vi "Save Para Setting UI.vi"() -> ()   [LabVIEW 2016]
uses:
  <vilib>/Utility/error.llb/DialogType.ctl
  Architecture/Queue Management/ARC_Queue Create_Single.vi
  Architecture/Queue Management/ARC_Queue Insert Element.vi
  Architecture/Queue Management/ARC_Queue Remove Element.vi
  Architecture/Queue Management/ARC_Queue Destroy_Single.vi
panel:
  in  "Parameter":cluster{"Q-Local":string, "Variant":variant}
  in  "Tab Control":enum32{"Page 1"}(tab)
  in  "AutoInterval":i32=1 caption="自动挑点时间间隔：" min=1 max=1000 step=1
  out "info":string
  in  "FileNote":string caption="文件备注："
  in  "FileName":string caption="文件名："
  in  "CFilePath":path caption="文件夹路径："
  in  "OK":bool
  out "error out":errorcluster caption="错误输出"
  # "文件存储设置"
  # "s"
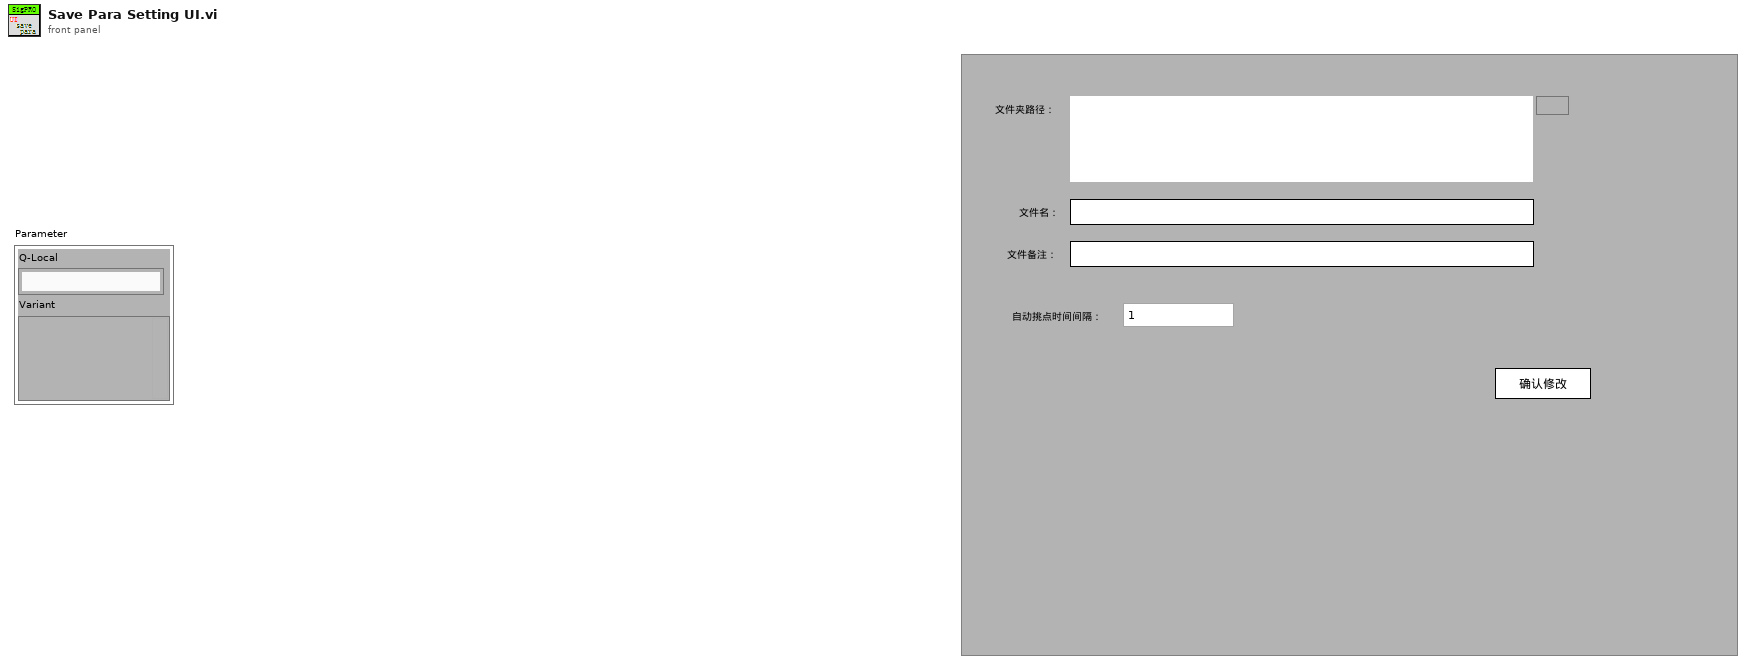
[diagram p1: front panel]
types:
  T1 = cluster{"error":errorcluster, "Event":string, "Data":variant, "Q_Local":string, "Caller":string, "Refs":cluster{"ContiousFileName":refnum<vi>, "SelectFileName":refnum<vi>, "CFilePath":refnum<vi>, "SFilePath":refnum<vi>}, "States":cluster{"CExist?":bool, "SExist?":bool}, "ContinuousFile？":bool}
  T2 = enum16{"open", "replace", "create", "open or create", "replace or create", "replace or create with confirmation"}
  T3 = typedef "DialogType.ctl" = u16
  T4 = typedef "Global para Config.ctl" = cluster{"Timing":cluster{"SampleRate":i32}, "SavePara":cluster{"FlowDiskMode":T5, "SelectMode":T6, "FolderPath":path, "Filename":string, "FileNote":string, "AutoInterval":i32, "Template":path}, "ConfigDS Path*":path, "Tdms Ref*":refnum<k34>}
  T5 = typedef "File Save Mode.ctl" = i32
  T6 = typedef "Select Point Mode.ctl" = i32
  T7 = cluster{"DfltDataFolder":path, "ParaFolder":path, "SysCfg":path, "CHdef":path, "ModCfg":path, "DT Folder":path, "ErrorLog":path, "HBMlic":path, "HBMDriver":path}
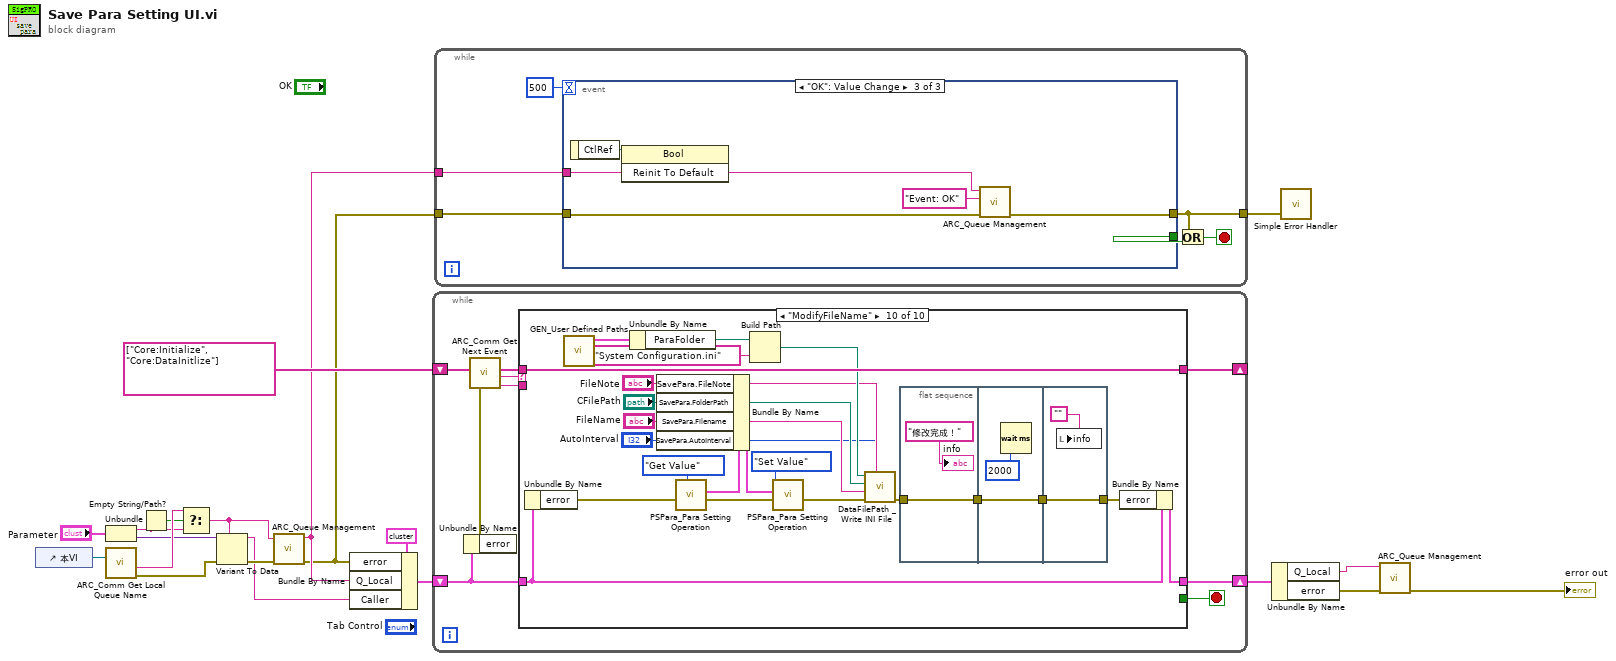
[diagram p0: block diagram]
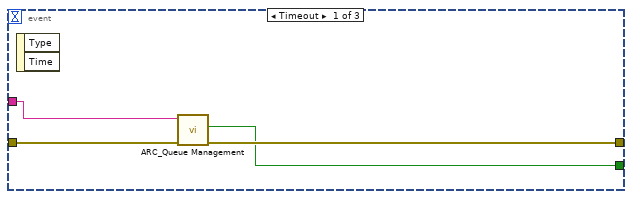
[diagram p2: hidden frame]
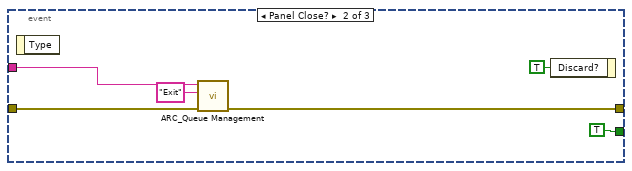
[diagram p3: hidden frame]
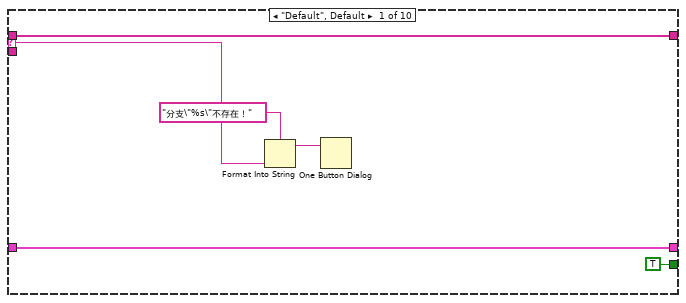
[diagram p4: hidden frame]
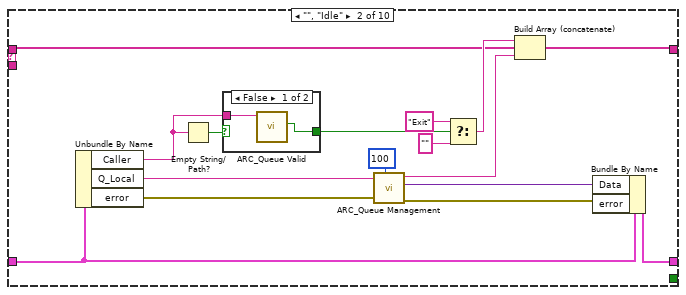
[diagram p5: hidden frame]
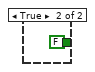
[diagram p6: hidden frame]
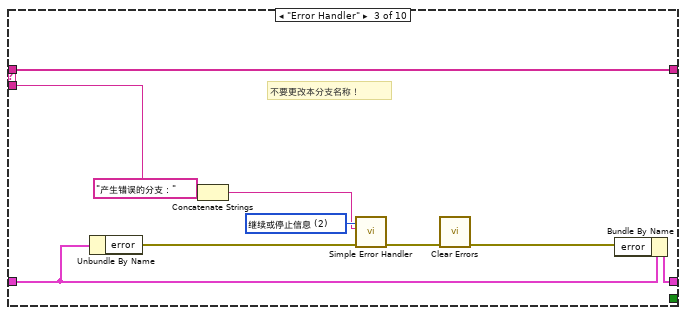
[diagram p7: hidden frame]
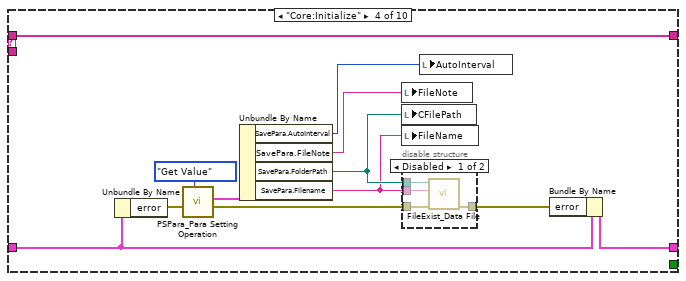
[diagram p8: hidden frame]
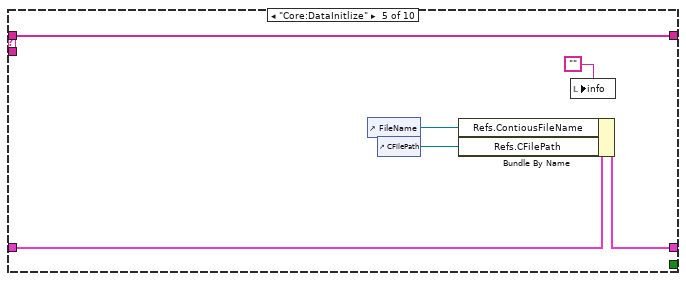
[diagram p10: hidden frame]
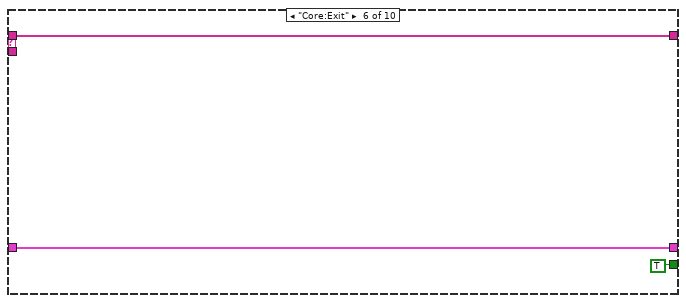
[diagram p11: hidden frame]
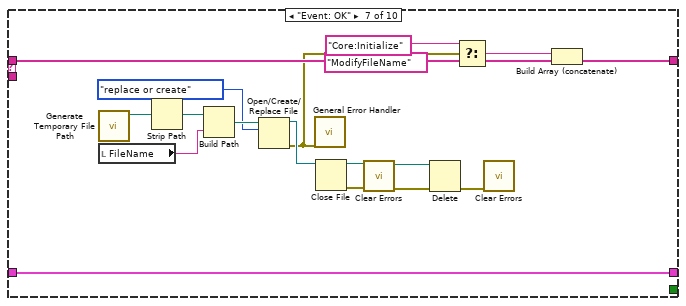
[diagram p12: hidden frame]
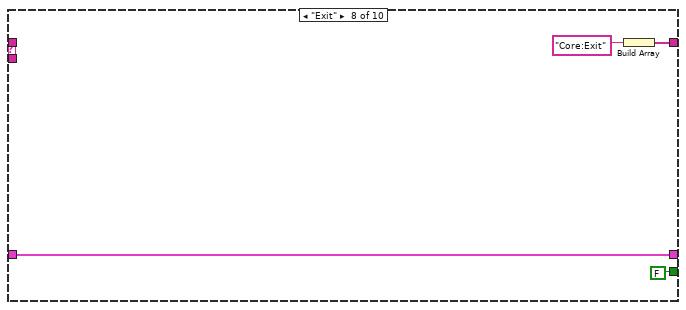
[diagram p13: hidden frame]
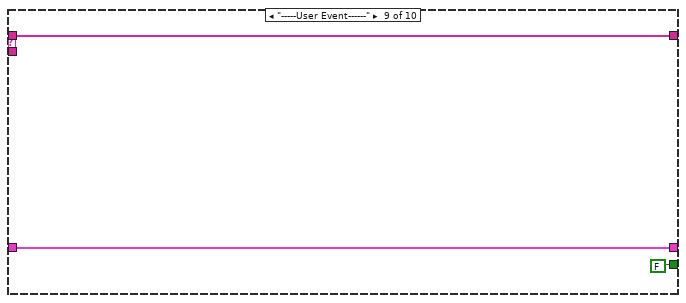
[diagram p14: hidden frame]
diagram:
  n1 = control-ref of="本VI"() -> (w6:refnum<vi>)
  n2 = Unbundle("Parameter") -> ("Q-Local"=w8:string, "Variant"=w11:variant)
  n3 = call "ARC_Comm Get Local Queue Name.vi"("VI Ref"=w6) -> ("error out"=w7:errorcluster, "VI  Name"=w12:string)  [unwired: 8 in, 1 out]
  n4 = Empty String/Path?(string/path=w8) -> (empty?=w10:bool)
  n5 = Select(t=w12, s=w10, f=w8) -> (s? t:f=w2:string)
  n6 = Variant To Data(error in=w7, type=w2, Variant=w11) -> (data=w1:string, error out=w5:errorcluster)
  n7 = call-poly "ARC_Queue Management.vi"("error in"=w5, "Queue Name"=w2) -> ("error out"=w3:errorcluster, "Queue Name dup"=w4:string)  [unwired: 7 in, 1 out]
  n8 = Bundle By Name(cluster=T1 {"error"={"status"=FALSE, "code"=0, "source"=""}, "Event"="", "Data"=variant, "Q_Local"="", "Caller"="", "Refs"={"ContiousFileName"=refnum, "SelectFileName"=refnum, "CFilePath"=refnum, "SFilePath"=refnum}, "States"={"CExist?"=FALSE, "SExist?"=FALSE}, "ContinuousFile？"=FALSE} ("TmpData"), "error"=w3, "Q_Local"=w4, "Caller"=w1) -> (w16:T1)
  n9 = while {
    shift-right: [w26] -> w19
    shift-left: w16 -> [w27]
    shift-right: [w25] -> _
    shift-left: string[] ["Core:Initialize", "Core:DataInitlize"] ("event queue out") -> [w21]
    stop <- w29 stop-if-true
    n10 = Unbundle By Name(w27) -> ("error"=w28:errorcluster)
    n11 = call "ARC_Comm Get Next Event.vi"("error in (no error)"=w28, "event queue in"=w21) -> ("prev event"=w24:string, "next event"=w22:string, "event queue out"=w23:string[])  [unwired: 4 in]
    n12 = case shown="\"ModifyFileName\"" w22 {
      selector: w22 -> [w33 _ _ _ _ _ _ _ _ _]
      tunnel: w23 -> [w34 w37 w64 w76 w87 w88 w106 _ w112 w132]
      tunnel: w24 -> [_ _ w55 _ _ _ _ _ _ _]
      tunnel: [TRUE _ _ _ _ TRUE _ FALSE FALSE _] -> w29
      tunnel: w27 -> [w35 w47 w60 w74 w86 w89 w107 w110 w113 w131]
      tunnel: [w35 w50 w59 w71 w85 w89 w107 w110 w113 w129] -> w26
      tunnel: [w34 w48 w64 w76 w87 w88 w105 w108 w112 w132] -> w25
      frame "Default", Default {
        n13 = Format Into String(format string="分支\"%s\"不存在！" ("格式字符串"), w33) -> (resulting string=w32:string)  [unwired: 2 in, 1 out]
        n14 = One Button Dialog(message=w32) -> ()  [unwired: 1 in, 1 out]
      }
      frame "", "Idle" {
        n15 = Unbundle By Name(w47) -> ("Caller"=w41:string, "Q_Local"=w46:string, "error"=w45:errorcluster)
        n16 = Empty String/Path?(string/path=w41) -> (empty?=w44:bool)
        n17 = case shown="False" w44 {
          tunnel: [w52 FALSE ("Not Exist?")] -> w43
          tunnel: w41 -> [w53 _]
          frame False {
            n18 = call "ARC_Queue Valid.vi"("Queue Name(unamed)"=w53) -> ("Not Exist?"=w52:bool)  [unwired: 8 in, 2 out]
          }
          frame True {
          }
        }
        n19 = call-poly "ARC_Queue Management.vi"("Time out(-1)_queue out"=100 ("Time out(-1)"), "error in (no error)"=w45, "Queue Name(unamed)"=w46) -> ("error out"=w51:errorcluster, "Data"=w49:variant, "Event"=w40:string)  [unwired: 5 in, 1 out]
        n20 = Select(t="Exit" ("Event"), s=w43, f="") -> (s? t:f=w38:string)
        n21 = Build Array (concatenate)(w38, w37, w40) -> (w48:string[])
        n22 = Bundle By Name(cluster=w47, "Data"=w49, "error"=w51) -> (w50:T1)
      }
      frame "Error Handler" {
        w58 = T3 2 items=["无对话框", "确定信息", "继续或停止信息", "确定信息＋警告", "继续/停止+警告"] ("type of dialog (OK msg:1)")
        # "不要更改本分支名称！"
        n23 = Unbundle By Name(w60) -> ("error"=w61:errorcluster)
        n24 = Concatenate Strings("产生错误的分支：" ("字符串"), w55) -> (w57:string)
        n25 = call <vilib>:"Simple Error Handler.vi"("error source (\" \")"=w57, "type of dialog (OK msg:1)"=w58, "error in (no error)"=w61) -> ("error out"=w62:errorcluster)  [unwired: 2 in, 4 out]
        n26 = call <vilib>:"Clear Errors.vi"("error in (no error)"=w62) -> ("error out"=w63:errorcluster)  [unwired: 5 in, 1 out]
        n27 = Bundle By Name(cluster=w60, "error"=w63) -> (w59:T1)
      }
      frame "Core:Initialize" {
        n28 = Unbundle By Name(w74) -> ("error"=w73:errorcluster)
        n29 = call "PSPara_Para Setting Operation.vi"("Operation"=enum16{"Set Value", "Get Value", "Initialize"}."Get Value", "error in"=w73) -> ("error out"=w70:errorcluster, "_Para"=w72:T4)  [unwired: 8 in]
        n30 = Unbundle By Name(w72) -> ("SavePara.AutoInterval"=w65:i32, "SavePara.FileNote"=w66:string, "SavePara.FolderPath"=w68:path, "SavePara.Filename"=w67:string)
        n31 = local write "FileNote"(w66) -> ()
        n32 = local write "CFilePath"(w68) -> ()
        n33 = local write "FileName"(w67) -> ()
        n34 = disable-structure shown="Disabled" {
          disable-tunnel: w70 -> [w80 w81]
          disable-tunnel: [w79 w81] -> w69
          disable-tunnel: w68 -> [w78 _]
          disable-tunnel: w67 -> [w77 _]
          frame Disabled {
            n35 = call "FileExist_Data File.vi"("error in"=w80, "Filename"=w77, "FolderPath"=w78) -> ("error out"=w79:errorcluster)  [unwired: 7 in, 1 out]
          }
          frame Enabled {
          }
        }
        n36 = local write "AutoInterval"(w65) -> ()
        n37 = Bundle By Name(cluster=w74, "error"=w69) -> (w71:T1)
      }
      frame "Core:DataInitlize" {
        n38 = control-ref of="FileName"() -> (w84:refnum<vi>)
        n39 = control-ref of="CFilePath"() -> (w83:refnum<vi>)
        n40 = Bundle By Name(cluster=w86, "Refs.ContiousFileName"=w84, "Refs.CFilePath"=w83) -> (w85:T1)
        n41 = local write "info"("") -> ()
      }
      frame "Core:Exit" {
      }
      frame "Event: OK" {
        n42 = call <vilib>:"Generate Temporary File Path.vi"() -> ("Unique Temporary File Path"=w101:path)  [unwired: 10 in, 1 out]
        n43 = local read "FileName"() -> (w104:string)
        n44 = Strip Path(path=w101) -> (stripped path=w91:path)  [unwired: 1 out]
        n45 = Build Path(base path=w91, name or relative path=w104) -> (appended path=w103:path)
        n46 = Open/Create/Replace File(file path (use dialog)=w103, operation (0:open)=T2."replace or create" ("操作(0:open)")) -> (refnum out=w100:refnum<file>, error out=w95:errorcluster)  [unwired: 4 in, 1 out]
        n47 = call <vilib>:"General Error Handler.vi"("error in (no error)"=w95) -> ()  [unwired: 10 in, 5 out]
        n48 = Close File(refnum=w100) -> (path=w99:path, error out=w98:errorcluster)  [unwired: 1 in]
        n49 = call <vilib>:"Clear Errors.vi"("error in (no error)"=w98) -> ("error out"=w97:errorcluster)  [unwired: 5 in, 1 out]
        n50 = Delete(path (use dialog)=w99, error in=w97) -> (error out=w96:errorcluster)  [unwired: 3 in, 2 out]
        n51 = Select(t="Core:Initialize", s=w95, f="ModifyFileName") -> (s? t:f=w92:string)
        n52 = call <vilib>:"Clear Errors.vi"("error in (no error)"=w96) -> ()  [unwired: 5 in, 2 out]
        n53 = Build Array (concatenate)(w92, w106) -> (w105:string[])
      }
      frame "Exit" {
        n54 = Build Array("Core:Exit" ("Remaining States")) -> (w108:string[])
      }
      frame "-----User Event------" {
      }
      frame "ModifyFileName" {
        n55 = Unbundle By Name(w131) -> ("error"=w130:errorcluster)
        n56 = call "GEN_User Defined Paths.vi"() -> ("UserDefinedPath"=w124:T7)  [unwired: 11 in]
        n57 = Unbundle By Name(w124) -> ("ParaFolder"=w123:path)
        n58 = call "PSPara_Para Setting Operation.vi"("Operation"=enum16{"Set Value", "Get Value", "Initialize"}."Get Value", "error in"=w130) -> ("error out"=w128:errorcluster, "_Para"=w134:T4)  [unwired: 8 in]
        n59 = Bundle By Name(cluster=w134, "SavePara.FileNote"="FileNote", "SavePara.FolderPath"="CFilePath", "SavePara.Filename"="FileName", "SavePara.AutoInterval"="AutoInterval") -> (w133:T4)
        n60 = Build Path(base path=w123, name or relative path="System Configuration.ini") -> (appended path=w121:path)
        n61 = call "PSPara_Para Setting Operation.vi"("Operation"=enum16{"Set Value", "Get Value", "Initialize"}."Set Value", "error in"=w128, "_Para"=w133) -> ("error out"=w127:errorcluster)  [unwired: 7 in, 1 out]
        n62 = call "DataFilePath _ Write INI File.vi"("AutoInterval"="AutoInterval", "FileNote"="FileNote", "error in"=w127, "FileName"="FileName", "DataFolder"="CFilePath", "INI File"=w121) -> ("error out"=w119:errorcluster)  [unwired: 5 in]
        n63 = flat-sequence {
          tunnel: w119 -> [w137]
          tunnel: [w137] -> w118
          tunnel: w118 -> [w140]
          tunnel: [w140] -> w117
          tunnel: [w142] -> w116
          tunnel: w117 -> [w142]
          frame #0 {
            "info" <- "修改完成！" ("消息")
          }
          frame #1 {
            n64 = Wait (ms)(milliseconds to wait=u32 2000 ("等待时间（毫秒）")) -> ()  [unwired: 1 out]
          }
          frame #2 {
            n65 = local write "info"("") -> ()
          }
        }
        n66 = Bundle By Name(cluster=w131, "error"=w116) -> (w129:T1)
      }
    }
  }
  n67 = while {
    tunnel: w3 -> [w147]
    tunnel: w4 -> [w148]
    tunnel: [w144] -> w18
    stop <- w145 stop-if-true
    n68 = event shown="[2] \"OK\": Value Change" {
      selector: _ -> [_ _ _]
      dyn-events: _ -> [_ _ _]
      timeout: 500 -> [_ _ _]
      tunnel: [w149 TRUE _] -> w146
      tunnel: w148 -> [w152 w157 w163]
      tunnel: w147 -> [w151 w156 w162]
      tunnel: [w150 w155 w160] -> w144
      event Timeout {
        n69 = event-data() -> ()  [unwired: 1 in, 2 out]
        n70 = call-poly "ARC_Queue Management.vi"("error in (no error)"=w151, "Queue Name(unamed)"=w152) -> ("error out"=w150:errorcluster, "Not Exist?"=w149:bool)  [unwired: 7 in, 1 out]
      }
      event Panel Close? {
        n71 = event-data() -> ()  [unwired: 1 in, 1 out]
        n72 = call-poly "ARC_Queue Management.vi"("error in (no error)"=w156, "Event"="Exit", "Queue Name(unamed)"=w157) -> ("error out"=w155:errorcluster)  [unwired: 7 in, 1 out]
        n73 = event-data("Discard?"=TRUE ("放弃？")) -> ()  [unwired: 1 in, 1 out]
      }
      event "OK": Value Change {
        n74 = event-data() -> ("CtlRef"=w159:refnum<vi>)  [unwired: 1 in]
        n75 = invoke class="Bool" method="Reinit To Default"(reference=w159) -> ()  [unwired: 2 in, 3 out]
        n76 = call-poly "ARC_Queue Management.vi"("error in (no error)"=w162, "Event"="Event: OK", "Queue Name(unamed)"=w163) -> ("error out"=w160:errorcluster)  [unwired: 7 in, 1 out]
      }
    }
    n77 = Or(x=w144, y=w146) -> (x .or. y?=w145:bool)
  }
  n78 = Unbundle By Name(w19) -> ("Q_Local"=w15:string, "error"=w20:errorcluster)
  n79 = call <vilib>:"Simple Error Handler.vi"("error in (no error)"=w18) -> ()  [unwired: 4 in, 5 out]
  n80 = call-poly "ARC_Queue Management.vi"("error in (no error)"=w20, "Queue Name(unamed)"=w15) -> ("error out"=→"error out":errorcluster)  [unwired: 7 in, 2 out]
